vi "SMGR File Viewer_Spectr_LF.vi"() -> ()   [LabVIEW 2010]
uses:
  <vilib>/Utility/miscctls.llb/LVRectTypeDef.ctl
  lib/Global 2.vi
  <vilib>/addons/Time Series Analysis/Correlation and Spectral Analysis.llb/TSA Cross-Correlation Function (Waveform).vi
  <vilib>/addons/_Advanced Signal Processing/NI_AdvSigProcTSA.lvlib
panel:
  in  "Tab Control":enum32{"signals", "spectra", "correlation"}(tab)
  out "i1":waveform(i16)[](graph) caption="KP-27"
  out "i2":waveform(i16)[](graph) caption="KP-27"
  in  "top":bool
  in  "bottom":bool
  out "Time Stamp":timestamp caption="t2" format="%<%.7X\n%x>T"
  out "Time Stamp 2":timestamp caption="t1" format="%<%.7X\n%x>T"
  out "x-y":dbl caption="t1-t2" format="%#_4p"
  in  "OK Button":bool
  out "x-y 2":dbl caption="С0-С1" format="%#_6p"
  out "x*y":dbl caption="Расстояние" format="%#_6p"
  in  "Boolean":bool caption="С фильтром"
  in  "Boolean 2":bool caption="С фильтром"
  out "Spectra":cluster{"f0":dbl, "df":dbl, "magnitude":dbl[]}[](graph)
  out "file path out":path
  out "correlogram":cluster{"Ramp Pattern":dbl[], "Rxy":dbl[]}(graph)
  out "cross-correlatuion":dbl[](graph)
  in  "cor":bool caption="вычисление кореляции"
  in  "index":i32
  in  "stop":bool
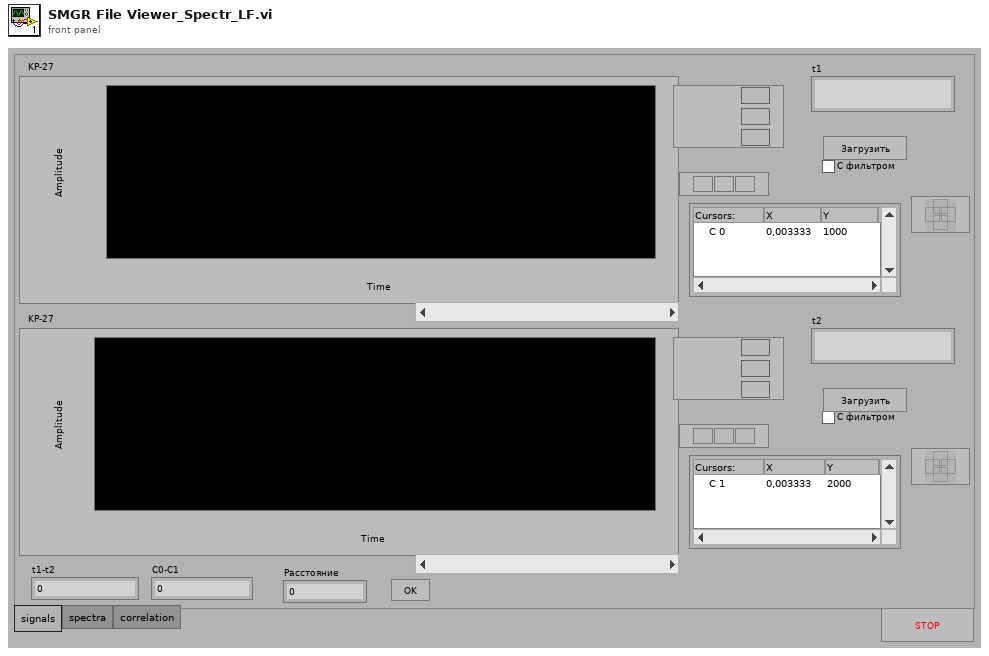
[diagram p1: front panel]
types:
  T1 = typedef "LVRectTypeDef.ctl" = cluster{"Left":i16, "Top":i16, "Right":i16, "Bottom":i16}
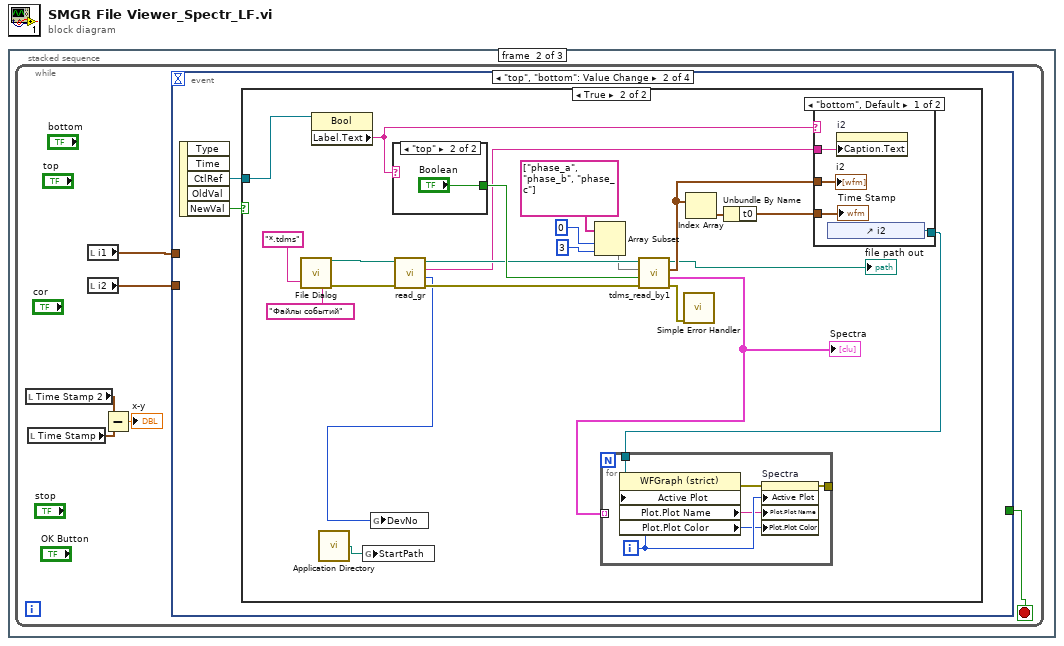
[diagram p0: block diagram]
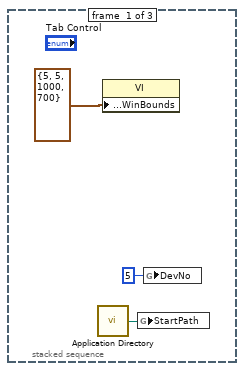
[diagram p2: hidden frame]
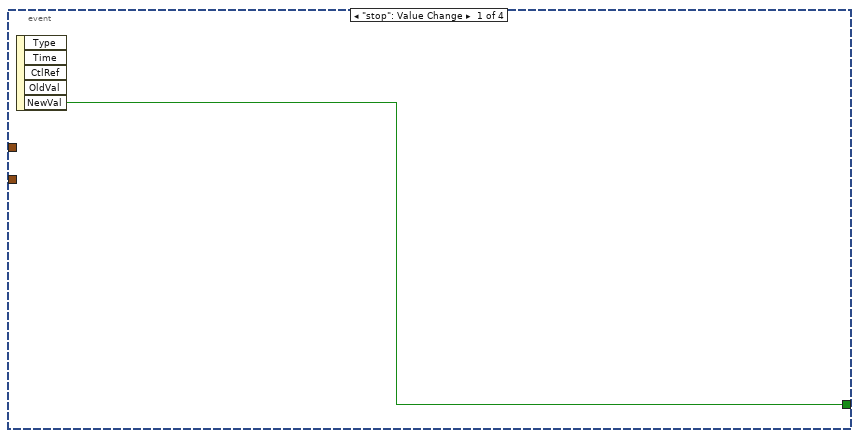
[diagram p3: hidden frame]
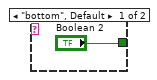
[diagram p5: hidden frame]
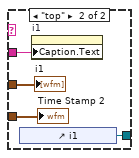
[diagram p6: hidden frame]
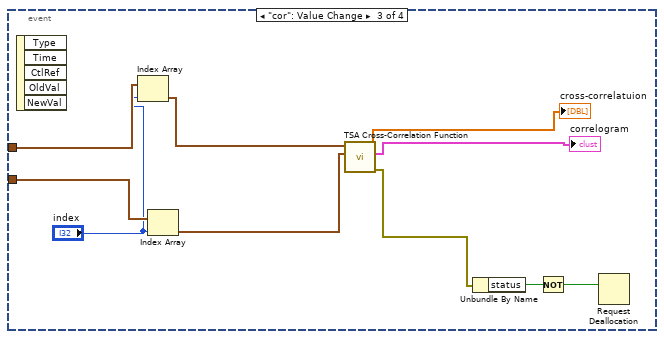
[diagram p7: hidden frame]
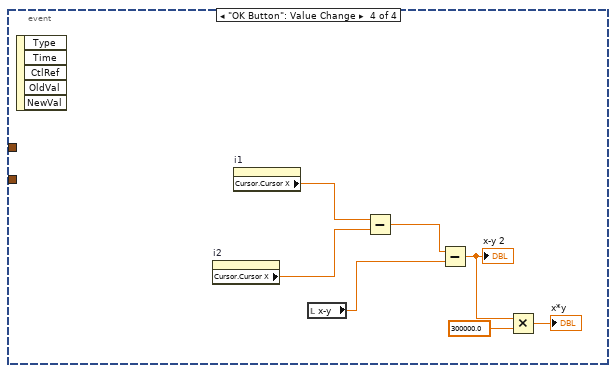
[diagram p8: hidden frame]
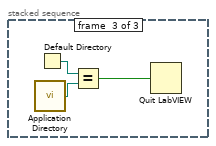
[diagram p9: hidden frame]
diagram:
  n1 = stacked-sequence {
    frame #0 {
      n2 = call <vilib>:"Application Directory.vi"() -> ("Application Directory"=w1:path)
      n3 = property on="Property Node" class="VI"("Front Panel.WinBounds"=T1 {"Left"=5, "Top"=5, "Right"=1000, "Bottom"=700} ("Front Panel Window:Panel Bounds")) -> ()  [unwired: 2 in, 2 out]
      n4 = global write "Global 2.vi" "StartPath"(w1) -> ()
      n5 = global write "Global 2.vi" "DevNo"(5 ("DevNo")) -> ()
    }
    frame #1 {
      n6 = while {
        stop <- w9 stop-if-true
        n7 = local read "Time Stamp 2"() -> (w6:timestamp)
        n8 = local read "Time Stamp"() -> (w7:timestamp)
        n9 = local read "i1"() -> (w5:waveform(i16)[])
        n10 = local read "i2"() -> (w4:waveform(i16)[])
        n11 = Subtract(x=w6, y=w7) -> (x-y=→"x-y":dbl)
        n12 = event shown="[1] \"top\", \"bottom\": Value Change" {
          selector: _ -> [_ _ _ _]
          dyn-events: _ -> [_ _ _ _]
          timeout: _ -> [_ _ _ _]
          tunnel: [w10 _ _ _] -> w9
          tunnel: w5 -> [_ _ w59 _]
          tunnel: w4 -> [_ _ w58 _]
          event "stop": Value Change {
            n13 = event-data() -> ("NewVal"=w10:bool)  [unwired: 1 in, 4 out]
          }
          event "top", "bottom": Value Change {
            n14 = event-data() -> ("CtlRef"=w11:refnum<vi>, "NewVal"=w12:bool)  [unwired: 1 in, 3 out]
            n15 = case shown="True" w12 {
              tunnel: w11 -> [_ w32]
              frame False {
              }
              frame True {
                n16 = call "File Dialog"("pattern (all files)"="*.tdms", "pattern label"="Файлы событий") -> ("selected path"=w22:path, "error out"=w21:errorcluster)  [unwired: 10 in, 2 out]
                n17 = property on="Property Node" class="Bool"(reference=w32) -> ("Label.Text"=w31:string)  [unwired: 1 in, 2 out]
                n18 = call <vilib>:"Application Directory.vi"() -> ("Application Directory"=w28:path)
                n19 = global write "Global 2.vi" "StartPath"(w28) -> ()
                n20 = case shown="\"top\"" w31 {
                  tunnel: ["Boolean 2" "Boolean"] -> w27
                  frame "bottom", Default {
                  }
                  frame "top" {
                  }
                }
                n21 = call "read_gr.vi"("error in"=w21, "datalog path"=w22) -> ("error out"=w19:errorcluster, "DevNo"=w18:i32, "group name"=w17:string, "new file path"=w20:path)  [unwired: 2 in]
                n22 = global write "Global 2.vi" "DevNo"(w18) -> ()
                n23 = Array Subset(array=string[] ["phase_a", "phase_b", "phase_c"], index=0, length=3) -> (w15:string[])
                n24 = call "tdms_read_by1.vi"("error in"=w19, "filter"=w27, "Array 3"=w15, "datalog path"=w20) -> ("error out"=w24:errorcluster, "Array 2"=w25:cluster{"f0":dbl, "df":dbl, "magnitude":dbl[]}[], "Array"=w26:waveform(i16)[], "file path out"=→"file path out":path)
                "Spectra" <- w25
                n25 = call <vilib>:"Simple Error Handler.vi"("error in (no error)"=w24) -> ()  [unwired: 4 in, 5 out]
                n26 = Index Array(array=w26) -> (element=w29:waveform(i16))  [unwired: 1 in]
                n27 = Unbundle By Name(w29) -> ("t0"=w33:timestamp)
                n28 = case shown="\"bottom\", Default" w31 {
                  tunnel: w26 -> [w46 w51]
                  tunnel: w33 -> [w47 w50]
                  tunnel: [w45 w49] -> w30
                  tunnel: w17 -> [w44 w48]
                  frame "bottom", Default {
                    n29 = control-ref of="i2"() -> (w45:refnum<vi>)
                    n30 = property on="i2" class="WFGraph (strict)"("Caption.Text"=w44) -> ()  [unwired: 2 in, 2 out]
                    "Time Stamp" <- w47
                    "i2" <- w46
                  }
                  frame "top" {
                    n31 = control-ref of="i1"() -> (w49:refnum<vi>)
                    n32 = property on="i1" class="WFGraph (strict)"("Caption.Text"=w48) -> ()  [unwired: 2 in, 2 out]
                    "i1" <- w51
                    "Time Stamp 2" <- w50
                  }
                }
                n33 = for {
                  tunnel: w30 -> [w38]
                  tunnel: [w36] -> _
                  tunnel: w25 -> [_] mode=indexing
                  i -> [w41]
                  n34 = property on="Property Node" class="WFGraph (strict)"(reference=w38, "Active Plot"=w41) -> (error out=w37:errorcluster, "Plot.Plot Name"=w40:string, "Plot.Plot Color"=w39:u32)  [unwired: 1 in, 1 out]
                  n35 = property on="Spectra" class="WFGraph (strict)"(error in=w37, "Active Plot"=w41, "Plot.Plot Name"=w40, "Plot.Plot Color"=w39) -> (error out=w36:errorcluster)  [unwired: 1 in, 1 out]
                }
              }
            }
          }
          event "cor": Value Change {
            n36 = event-data() -> ()  [unwired: 1 in, 5 out]
            n37 = Index Array(array=w59, index="index") -> (element=w56:waveform(i16))
            n38 = Index Array(array=w58, index="index") -> (element=w57:waveform(i16))
            n39 = call-poly <vilib>:"TSA Cross-Correlation Function.vi"("Yt"=w57, "Xt"=w56) -> ("error out"=w54:errorcluster, "correlogram"=→"correlogram":cluster{"Ramp Pattern":dbl[], "Rxy":dbl[]}, "cross-correlation"=→"cross-correlatuion":dbl[])  [unwired: 7 in]
            n40 = Unbundle By Name(w54) -> ("status"=w53:bool)
            n41 = Not(x=w53) -> (.not. x?=w52:bool)
            n42 = Request Deallocation(w52) -> ()
          }
          event "OK Button": Value Change {
            n43 = event-data() -> ()  [unwired: 1 in, 5 out]
            n44 = property on="i2" class="WFGraph (strict)"() -> ("Cursor.Cursor X"=w62:dbl)  [unwired: 2 in, 2 out]
            n45 = property on="i1" class="WFGraph (strict)"() -> ("Cursor.Cursor X"=w63:dbl)  [unwired: 2 in, 2 out]
            n46 = local read "x-y"() -> (w67:dbl)
            n47 = Subtract(x=w63, y=w62) -> (x-y=w68:dbl)
            n48 = Subtract(x=w68, y=w67) -> (x-y=w66:dbl)
            "x-y 2" <- w66
            n49 = Multiply(x=w66, y=300000.0) -> (x*y=→"x*y":dbl)
          }
        }
      }
    }
    frame #2 {
      n50 = call <vilib>:"Application Directory.vi"() -> ("Application Directory"=w70:path)
      n51 = Default Directory() -> (w71:path)
      n52 = Equal?(x=w71, y=w70) -> (x = y?=w69:bool)
      n53 = Quit LabVIEW(quit? (T)=w69) -> ()
    }
  }
